vi "counter-i.vi"(7 "init ?":bool, 10 "cricket interval":i32=-1) -> (2 "cricket":bool=TRUE, 3 "tic":i32)   [LabVIEW 2015]
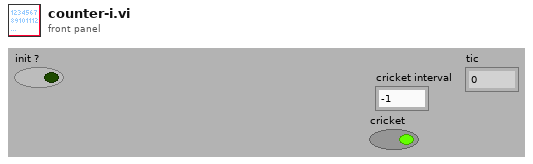
[diagram p1: front panel]
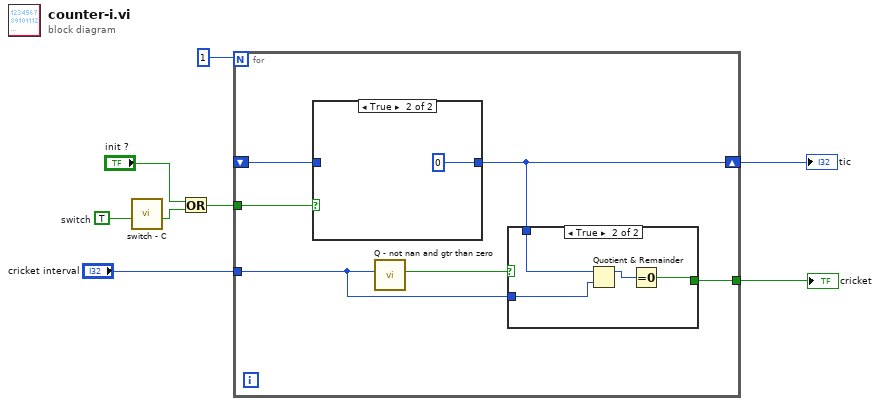
[diagram p0: block diagram]
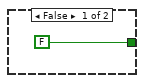
[diagram p2: hidden frame]
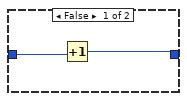
[diagram p3: hidden frame]
diagram:
  w7 = TRUE  # switch
  n1 = call "switch - C.vi"("switch"=w7) -> ("result"=w3:bool)  [unwired: 10 in]
  n2 = Or(x="init ?", y=w3) -> (x .or. y?=w1:bool)
  n3 = for {
    N: 1 -> [_]
    tunnel: w1 -> [w14]
    shift-right: [w10] -> w4
    shift-left: _ -> [w13]
    tunnel: "cricket interval" -> [w9]
    tunnel: [w11] -> w5
    n4 = case shown="True" w14 {
      tunnel: [w20 0] -> w10
      tunnel: w13 -> [w21 _]
      frame False {
        n5 = Increment(x=w21) -> (x+1=w20:i32)
      }
      frame True {
      }
    }
    n6 = call "Q - not nan and gtr than zero.vi"("Numeric"=w9) -> ("Boolean"=w12:bool)  [unwired: 10 in]
    n7 = case shown="True" w12 {
      tunnel: [FALSE w16] -> w11
      tunnel: w10 -> [_ w19]
      tunnel: w9 -> [_ w18]
      frame False {
      }
      frame True {
        n8 = Quotient & Remainder(x=w19, y=w18) -> (x-y*floor(x/y)=w17:i32)  [unwired: 1 out]
        n9 = Equal To 0?(x=w17) -> (x = 0?=w16:bool)
      }
    }
  }
  "cricket" <- w5
  "tic" <- w4
